vi "ReadBoolean.vi"(1 "reference":refnum<k24>, 2 "symbolPath":string) -> (0 "output":bool)   [LabVIEW 2020]
uses:
  C:/TwinCAT/AdsApi/.NET/v4.0.30319/TwinCAT.Ads.dll
  TwinCAT/AdsApi/.NET/v4.0.30319/TwinCAT.Ads.dll
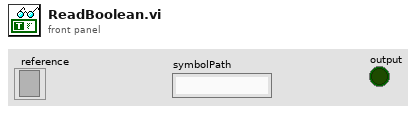
[diagram p1: front panel]
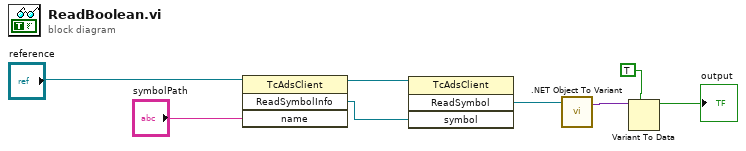
[diagram p0: block diagram]
diagram:
  n1 = invoke class="TcAdsClient" method="ReadSymbolInfo"(reference="reference", "name"="symbolPath") -> (reference out=w8:refnum<k24>, "ReadSymbolInfo"=w7:refnum<k24>)  [unwired: 2 in, 2 out]
  n2 = invoke class="TcAdsClient" method="ReadSymbol"(reference=w8, "symbol"=w7) -> ("ReadSymbol"=w6:refnum<k24>)  [unwired: 2 in, 3 out]
  n3 = call <vilib>:".NET Object To Variant.vi"(".NET object"=w6) -> ("variant"=w5:variant)  [unwired: 1 in, 1 out]
  n4 = Variant To Data(type=TRUE, Variant=w5) -> (data=→"output":bool)  [unwired: 1 in, 1 out]
